vi "Write Main CD Properties.vi"(8 "error in (no error)":errorcluster, 10 "Main CD Properties":T1, 11 "CustomDeviceRepo in":refnum<class "CustomDeviceRepo.lvclass">) -> (0 "error out":errorcluster, 3 "CustomDeviceRepo out":refnum<class "CustomDeviceRepo.lvclass">)   [LabVIEW 2019, in "CustomDeviceRepo.lvclass"]
uses:
  CustomDeviceRepo.lvclass
  XML Controls/Main Custom Device Properties.ctl
  CustomDeviceRepo.lvclass/CustomDeviceRepo.ctl
  VeriStand Custom Device XML Parser.lvlib
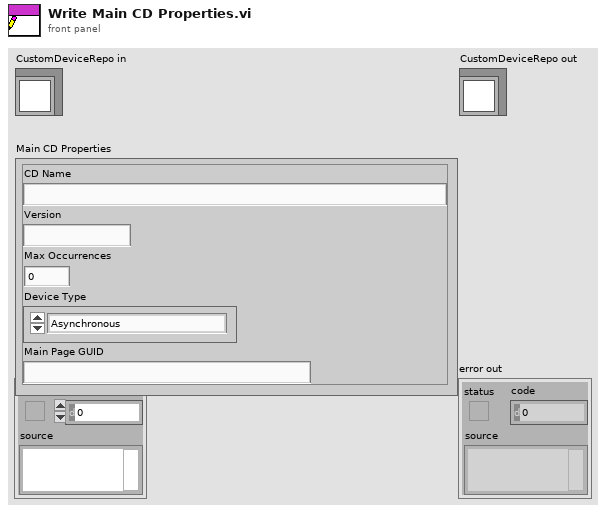
[diagram p1: front panel]
types:
  T1 = typedef "VeriStand Custom Device XML Parser.lvlib/Main Custom Device Properties.ctl" = cluster{"CD Name":string, "Version":string, "Max Occurrences":i32, "Device Type":enum16{"Asynchronous", "Inline HW Interface", "Inline Model Interface", "Inline Timing and Sync", "Asynchronous Timing and Sync"}, "Main Page GUID":string}
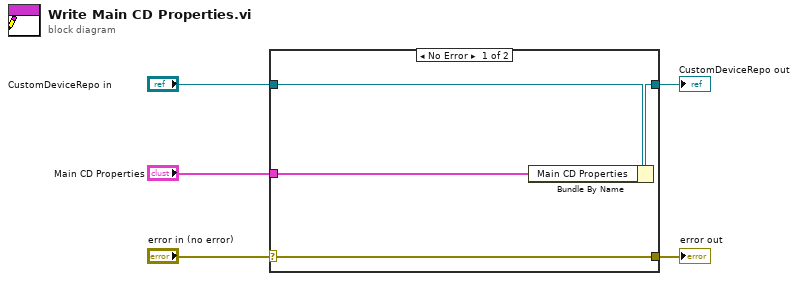
[diagram p0: block diagram]
diagram:
  n1 = case shown="No Error" "error in (no error)" {
    selector: "error in (no error)" -> [w9 w10]
    tunnel: [w9 w10] -> w4
    tunnel: [w7 w11] -> w2
    tunnel: "CustomDeviceRepo in" -> [w8 w11]
    tunnel: "Main CD Properties" -> [w6 _]
    frame No Error {
      n2 = Bundle By Name(cluster=w8, "Main CD Properties"=w6) -> (w7:refnum<class "CustomDeviceRepo.lvclass">)
    }
    frame Error {
    }
  }
  "error out" <- w4
  "CustomDeviceRepo out" <- w2
